vi "Add Arc to Exit.vi"(6 "Tangent Start Angle (rad)":dbl, 7 "Dist per Points":dbl=3000.0, 8 "Additional circle arc (rad)":dbl, 9 "Tangent Point":cluster{dbl, dbl}, 10 "Radius":dbl, 11 "Center Point":cluster{dbl, dbl}) -> (1 "Point Arrays":cluster{dbl[], dbl[], dbl[]}, 2 "Arc Distance":dbl, 3 "Blend Exit Point":cluster{dbl, dbl})   [LabVIEW 2025]
panel:
  out "Array":dbl[](array[numeric])
  out "Waveform Graph":dbl[](graph)
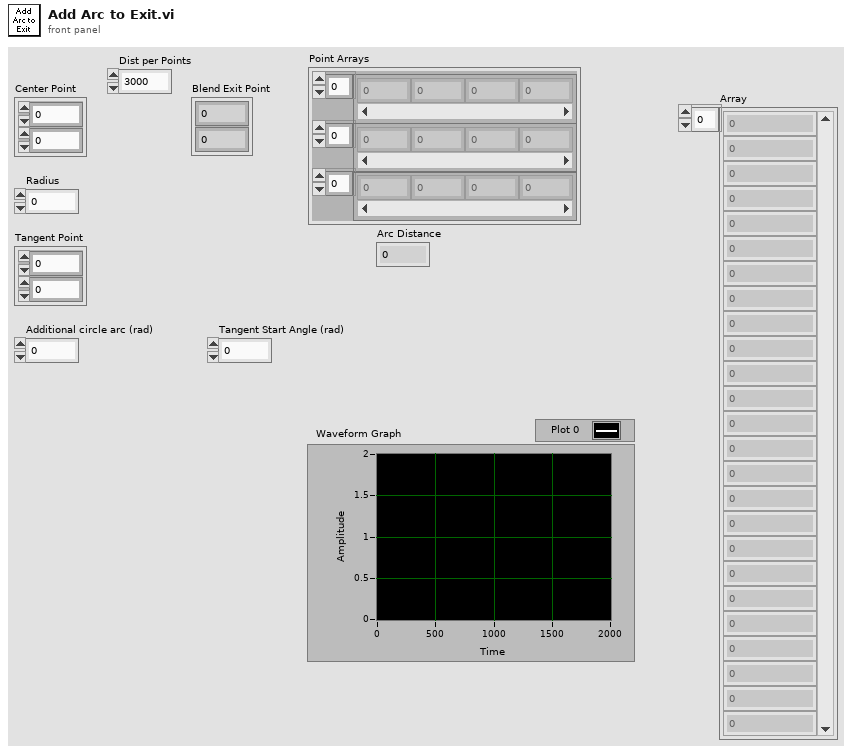
[diagram p1: front panel]
types:
  T1 = cluster{"appended array":dbl[], "appended array":dbl[], "appended array":dbl[]}
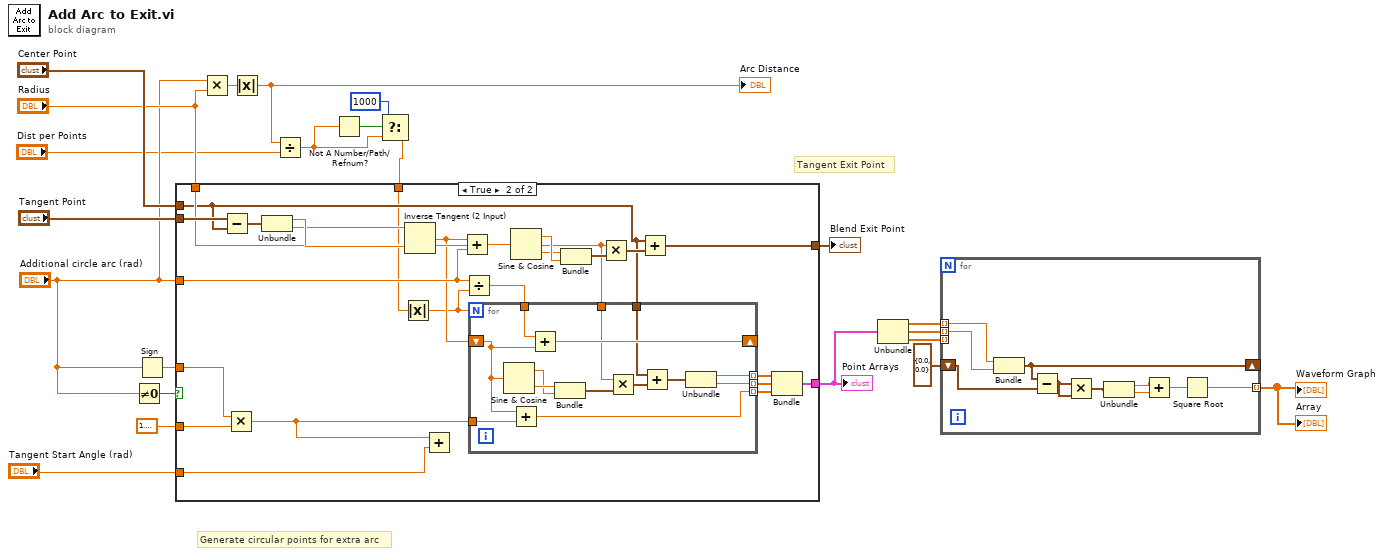
[diagram p0: block diagram]
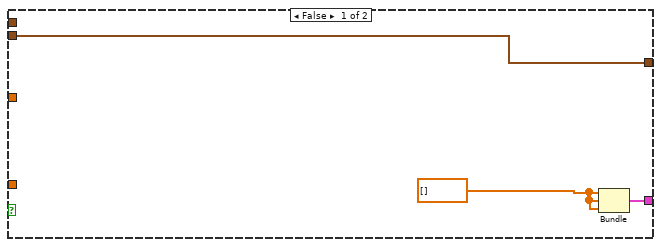
[diagram p2: hidden frame]
diagram:
  # "Generate circular points for extra arc"
  # "Tangent Exit Point"
  n1 = Not Equal To 0?(x="Additional circle arc (rad)") -> (x != 0?=w19:bool)
  n2 = Sign(1:"Additional circle arc (rad)") -> (0:w18:dbl)
  n3 = Multiply(x="Additional circle arc (rad)", y="Radius") -> (x*y=w13:dbl)
  n4 = Absolute Value(x=w13) -> (abs(x)=w12:dbl)
  "Arc Distance" <- w12
  n5 = Divide(x=w12, y="Dist per Points") -> (x/y=w9:dbl)
  n6 = Not A Number/Path/Refnum?(number/path/refnum=w9) -> (NaN/Path/Refnum?=w10:bool)
  n7 = Select(t=1000, s=w10, f=w9) -> (s? t:f=w8:dbl)
  n8 = case shown="True" w19 {
    tunnel: [w25 w50] -> w22
    tunnel: "Tangent Point" -> [w25 w42]
    tunnel: "Additional circle arc (rad)" -> [_ w40]
    tunnel: "Radius" -> [_ w38]
    tunnel: "Center Point" -> [_ w37]
    tunnel: [w24 w34] -> w2
    tunnel: w18 -> [_ w32]
    tunnel: 1.5707963267948966 -> [_ w31]
    tunnel: "Tangent Start Angle (rad)" -> [_ w29]
    tunnel: w8 -> [_ w27]
    frame False {
      w23 = dbl[] [] ("appended array")
      n9 = Bundle("appended array"=w23, "appended array"=w23, "appended array"=w23) -> (w24:T1)  [unwired: 1 in]
    }
    frame True {
      n10 = Subtract(x=w42, y=w37) -> (x-y=w43:cluster{dbl, dbl})
      n11 = Multiply(x=w32, y=w31) -> (x*y=w28:dbl)
      n12 = Unbundle(w43) -> (w45:dbl, w44:dbl)
      n13 = Absolute Value(x=w27) -> (abs(x)=w26:dbl)
      n14 = Inverse Tangent (2 Input)(1:w45, 2:w44) -> (0:w30:dbl)
      n15 = Add(x=w28, y=w29) -> ()  [unwired: 1 out]
      n16 = Add(x=w30, y=w40) -> (x+y=w41:dbl)
      n17 = Divide(x=w40, y=w26) -> (x/y=w39:dbl)
      n18 = for {
        N: w26 -> [_]
        shift-right: [w62] -> _
        shift-left: w30 -> [w52]
        tunnel: w39 -> [w61]
        tunnel: w37 -> [w59]
        tunnel: w38 -> [w58]
        tunnel: [w55] -> w36 mode=indexing
        tunnel: [w54] -> w35 mode=indexing
        tunnel: [w51] -> w33 mode=indexing
        tunnel: w28 -> [w53]
        n19 = Sine & Cosine(0:w52) -> (1:w63:dbl, 2:w64:dbl)
        n20 = Add(x=w52, y=w53) -> (x+y=w51:dbl)
        n21 = Add(x=w61, y=w52) -> (x+y=w62:dbl)
        n22 = Bundle(w64, w63) -> (w57:cluster{dbl, dbl})  [unwired: 1 in]
        n23 = Multiply(x=w58, y=w57) -> (x*y=w60:cluster{dbl, dbl})
        n24 = Add(x=w59, y=w60) -> (x+y=w56:cluster{dbl, dbl})
        n25 = Unbundle(w56) -> (w55:dbl, w54:dbl)
      }
      n26 = Sine & Cosine(0:w41) -> (1:w47:dbl, 2:w46:dbl)
      n27 = Bundle(w46, w47) -> (w48:cluster{dbl, dbl})  [unwired: 1 in]
      n28 = Multiply(x=w38, y=w48) -> (x*y=w49:cluster{dbl, dbl})
      n29 = Add(x=w37, y=w49) -> (x+y=w50:cluster{dbl, dbl})
      n30 = Bundle(w36, w35, w33) -> (w34:cluster{dbl[], dbl[], dbl[]})  [unwired: 1 in]
    }
  }
  "Blend Exit Point" <- w22
  "Point Arrays" <- w2
  n31 = Unbundle(w2) -> ("appended array"=w6:dbl[], "appended array"=w5:dbl[], "appended array"=w4:dbl[])
  n32 = for {
    tunnel: w6 -> [w74] mode=indexing
    tunnel: w5 -> [w73] mode=indexing
    tunnel: w4 -> [_] mode=indexing
    shift-right: [w72] -> _
    shift-left: cluster{dbl, dbl} {0.0, 0.0} -> [w71]
    tunnel: [w65] -> w1 mode=indexing
    n33 = Bundle(w74, w73) -> (w72:cluster{dbl, dbl})  [unwired: 1 in]
    n34 = Subtract(x=w72, y=w71) -> (x-y=w70:cluster{dbl, dbl})
    n35 = Multiply(x=w70, y=w70) -> (x*y=w69:cluster{dbl, dbl})
    n36 = Unbundle(w69) -> (w68:dbl, w67:dbl)
    n37 = Add(x=w68, y=w67) -> (x+y=w66:dbl)
    n38 = Square Root(x=w66) -> (sqrt(x)=w65:dbl)
  }
  "Waveform Graph" <- w1
  "Array" <- w1
